vi "TriWave2ndEd_YNWang.vi"() -> ()   [LabVIEW 2014]
uses:
  <vilib>/Instr/_visa.llb/VISA Configure Serial Port (Instr).vi
panel:
  out "Measured Curr":dbl
  out "Output Volt":dbl
  out "V-I Diagram":cluster{dbl[], dbl[]}(graph)
  in  "VISA Name":refnum<visa-resource-name>
  in  "Path":path
  in  "Protect Scan":bool
  in  "Reverse?":bool
  in  "Pause":bool
  in  "stop":bool
  in  "End":dbl format="%#_13g"
  in  "Cycle":i32
  in  "milliseconds to wait":u32
  out "Output V":dbl(graph)
  in  "Init":dbl format="%#_13g"
  in  "step":dbl format="%#_13g"
  in  "Min":dbl format="%#_13g"
  in  "Max":dbl format="%#_13g"
  # "Reverse"
  # "Normal"
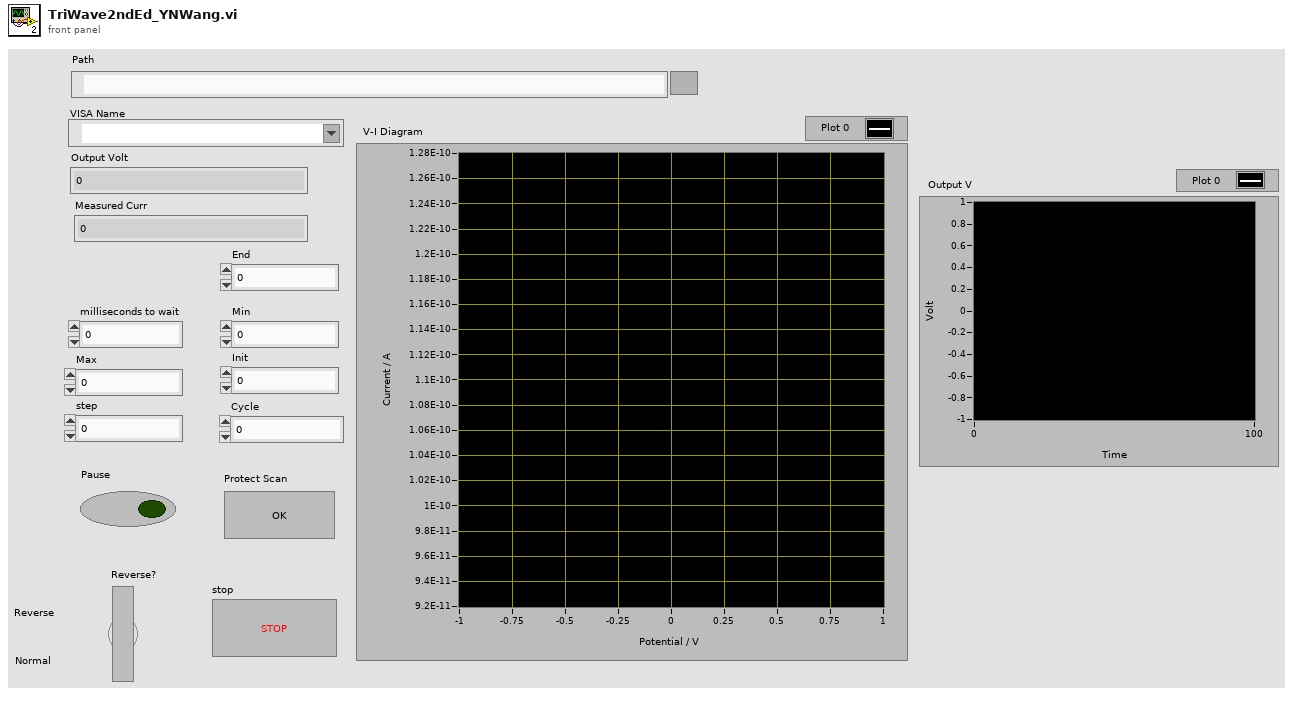
[diagram p1: front panel]
types:
  T1 = enum16{"open", "replace", "create", "open or create", "replace or create", "replace or create with confirmation"}
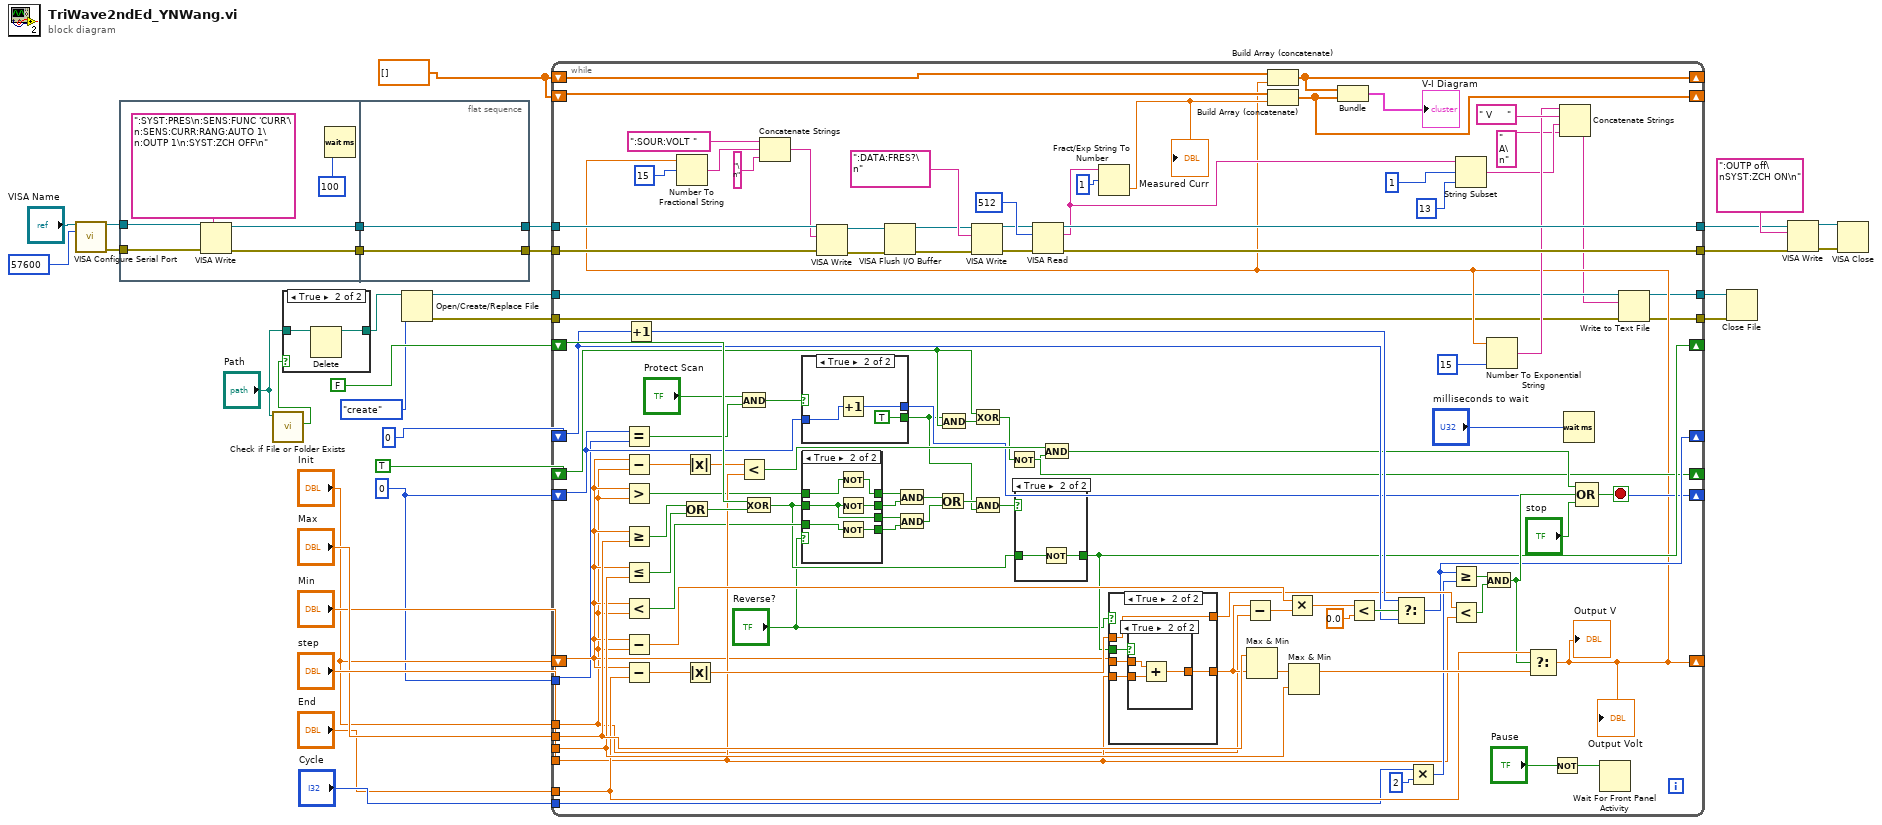
[diagram p0: block diagram]
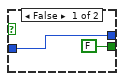
[diagram p3: hidden frame]
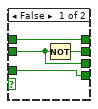
[diagram p4: hidden frame]
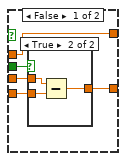
[diagram p6: hidden frame]
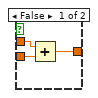
[diagram p7: hidden frame]
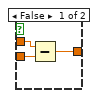
[diagram p8: hidden frame]
diagram:
  w16 = dbl[] []
  w24 = 0
  n1 = call-poly "VISA Configure Serial Port"("VISA resource name"="VISA Name", "baud rate (9600)"=57600) -> ("VISA resource name out"=w13:refnum<visa-resource-name>, "error out"=w12:errorcluster)  [unwired: 12 in]
  n2 = flat-sequence {
    tunnel: w13 -> [w38]
    tunnel: w12 -> [w37]
    tunnel: [w34] -> w4
    tunnel: [w33] -> w3
    tunnel: [w39] -> w1
    tunnel: [w40] -> w2
    tunnel: w4 -> [w40]
    tunnel: w3 -> [w39]
    frame #0 {
      n3 = VISA Write(VISA resource name=w38, write buffer=":SYST:PRES\n:SENS:FUNC 'CURR'\n:SENS:CURR:RANG:AUTO 1\n:OUTP 1\n:SYST:ZCH OFF\n", error in (no error)=w37) -> (VISA resource name out=w34:refnum<visa-resource-name>, error out=w33:errorcluster)  [unwired: 1 out]
      n4 = Wait (ms)(milliseconds to wait=u32 100) -> ()  [unwired: 1 out]
    }
    frame #1 {
    }
  }
  n5 = call <vilib>:"Check if File or Folder Exists.vi"("path"="Path") -> ("file or folder exists?"=w22:bool)  [unwired: 8 in, 2 out]
  n6 = case shown="True" w22 {
    tunnel: "Path" -> [w41 w43]
    tunnel: [w41 w42] -> w20
    frame False {
    }
    frame True {
      n7 = Delete(path (use dialog)=w43) -> (deleted path=w42:path)  [unwired: 4 in, 2 out]
    }
  }
  n8 = Open/Create/Replace File(file path (use dialog)=w20, operation (0:open)=T1."create") -> (refnum out=w18:refnum<file>, error out=w17:errorcluster)  [unwired: 4 in, 1 out]
  n9 = while {
    tunnel: "step" -> [w109]
    tunnel: "Max" -> [w139]
    tunnel: "Min" -> [w137]
    shift-right: [w112] -> _
    shift-left: FALSE -> [w142]
    shift-right: [w55] -> _
    shift-left: "Init" -> [w105]
    tunnel: "Init" -> [w104]
    shift-right: [w115] -> _
    shift-left: 0 -> [w129]
    tunnel: "Cycle" -> [w119]
    tunnel: "End" -> [w123]
    tunnel: w24 -> [w93]
    shift-right: [w95] -> _
    shift-left: w24 -> [w94]
    shift-right: [w87] -> _
    shift-left: TRUE -> [w88]
    tunnel: w18 -> [w54]
    tunnel: w17 -> [w53]
    tunnel: w2 -> [w75]
    tunnel: w1 -> [w74]
    tunnel: [w65] -> w8
    tunnel: [w64] -> w7
    tunnel: [w51] -> w6
    tunnel: [w50] -> w5
    shift-right: [w49] -> _
    shift-left: w16 -> [w81]
    shift-right: [w48] -> _
    shift-left: w16 -> [w80]
    stop <- w120 stop-if-true
    n10 = Equal?(x=w94, y=w93) -> (x = y?=w90:bool)
    n11 = Subtract(x=w105, y=w104) -> (x-y=w111:dbl)
    n12 = Greater?(x=w105, y=w104) -> (0:w100:bool)
    n13 = Greater Or Equal?(x=w105, y=w139) -> (x >= y?=w144:bool)
    n14 = Less Or Equal?(x=w105, y=w137) -> (x <= y?=w143:bool)
    n15 = Less?(x=w105, y=w104) -> (x < y?=w101:bool)
    n16 = Subtract(x=w105, y=w104) -> (x-y=w134:dbl)
    n17 = Subtract(x=w105, y=w123) -> (x-y=w128:dbl)
    n18 = Increment(x=w129) -> (x+1=w130:i32)
    n19 = Or(x=w144, y=w143) -> (x .or. y?=w141:bool)
    n20 = Absolute Value(x=w111) -> (abs(x)=w110:dbl)
    n21 = Absolute Value(x=w128) -> (abs(x)=w127:dbl)
    n22 = And(x="Protect Scan", y=w90) -> (x .and. y?=w92:bool)
    n23 = Less?(x=w110, y=w109) -> (x < y?=w108:bool)
    n24 = Exclusive Or(1:w141, 2:w142) -> (0:w98:bool)
    n25 = case shown="True" w92 {
      tunnel: [FALSE TRUE] -> w85
      tunnel: w94 -> [w145 w148]
      tunnel: [w145 w147] -> w95
      frame False {
      }
      frame True {
        n26 = Increment(x=w148) -> (x+1=w147:i32)
      }
    }
    n27 = case shown="True" "Reverse?" {
      tunnel: w101 -> [w152 w157]
      tunnel: w98 -> [w150 w154]
      tunnel: w100 -> [w153 w159]
      tunnel: [w153 w158] -> w99
      tunnel: [w152 w156] -> w83
      tunnel: [w150 w154] -> w84
      tunnel: [w151 w155] -> w82
      frame False {
        n28 = Not(x=w150) -> (.not. x?=w151:bool)
      }
      frame True {
        n29 = Not(x=w159) -> (.not. x?=w158:bool)
        n30 = Not(x=w154) -> (.not. x?=w155:bool)
        n31 = Not(x=w157) -> (.not. x?=w156:bool)
      }
    }
    n32 = And(x=w99, y=w82) -> (x .and. y?=w106:bool)
    n33 = And(x=w84, y=w83) -> (x .and. y?=w103:bool)
    n34 = Or(x=w106, y=w103) -> (x .or. y?=w97:bool)
    n35 = And(x=w85, y=w88) -> (x .and. y?=w89:bool)
    n36 = Exclusive Or(1:w89, 2:w88) -> (0:w87:bool)
    n37 = And(x=w97, y=w85) -> (x .and. y?=w102:bool)
    n38 = Not(x=w87) -> (.not. x?=w86:bool)
    n39 = case shown="True" w102 {
      tunnel: w98 -> [w160 w161]
      tunnel: [w160 w162] -> w112
      frame False {
      }
      frame True {
        n40 = Not(x=w161) -> (.not. x?=w162:bool)
      }
    }
    n41 = And(x=w108, y=w86) -> (x .and. y?=w107:bool)
    n42 = case shown="True" "Reverse?" {
      tunnel: w109 -> [w165 w176]
      tunnel: w105 -> [w166 w177]
      tunnel: [w164 w175] -> w136
      tunnel: w127 -> [w163 w174]
      tunnel: [w163 w174] -> w126
      tunnel: w112 -> [w167 w178]
      frame False {
        n43 = case shown="True" w167 {
          tunnel: w166 -> [w170 w173]
          tunnel: w165 -> [w169 w172]
          tunnel: [w168 w171] -> w164
          frame False {
            n44 = Add(x=w170, y=w169) -> (x+y=w168:dbl)
          }
          frame True {
            n45 = Subtract(x=w173, y=w172) -> (x-y=w171:dbl)
          }
        }
      }
      frame True {
        n46 = case shown="True" w178 {
          tunnel: w177 -> [w181 w184]
          tunnel: w176 -> [w180 w183]
          tunnel: [w179 w182] -> w175
          frame False {
            n47 = Subtract(x=w181, y=w180) -> (x-y=w179:dbl)
          }
          frame True {
            n48 = Add(x=w184, y=w183) -> (x+y=w182:dbl)
          }
        }
      }
    }
    n49 = Subtract(x=w136, y=w104) -> (x-y=w135:dbl)
    n50 = Max & Min(x=w139, y=w136) -> (min(x,y)=w138:dbl)  [unwired: 1 out]
    n51 = Multiply(x=w134, y=w135) -> (x*y=w133:dbl)
    n52 = Max & Min(x=w138, y=w137) -> (max(x,y)=w124:dbl)  [unwired: 1 out]
    n53 = Less?(x=w133, y=0.0) -> (x < y?=w131:bool)
    n54 = Select(t=w130, s=w131, f=w129) -> (s? t:f=w115:i32)
    n55 = Multiply(x=w119, y=2) -> (x*y=w116:i32)
    n56 = Greater Or Equal?(x=w115, y=w116) -> (x >= y?=w117:bool)
    n57 = Less?(x=w126, y=w109) -> (x < y?=w125:bool)
    n58 = And(x=w117, y=w125) -> (x .and. y?=w121:bool)
    n59 = Select(t=w123, s=w121, f=w124) -> (s? t:f=w55:dbl)
    "Output V" <- w55
    "Output Volt" <- w55
    n60 = Number To Fractional String(number=w55, width (-)=15) -> (F-format string=w77:string)  [unwired: 2 in]
    n61 = Concatenate Strings(":SOUR:VOLT ", w77, "\n") -> (w73:string)
    n62 = VISA Write(VISA resource name=w75, write buffer=w73, error in (no error)=w74) -> (VISA resource name out=w47:refnum<visa-resource-name>, error out=w46:errorcluster)  [unwired: 1 out]
    n63 = VISA Flush I/O Buffer(VISA resource name=w47, error in (no error)=w46) -> (VISA resource name out=w45:refnum<visa-resource-name>, error out=w44:errorcluster)  [unwired: 1 in]
    n64 = VISA Write(VISA resource name=w45, write buffer=":DATA:FRES?\n", error in (no error)=w44) -> (VISA resource name out=w69:refnum<visa-resource-name>, error out=w68:errorcluster)  [unwired: 1 out]
    n65 = VISA Read(VISA resource name=w69, byte count=u32 512, error in (no error)=w68) -> (VISA resource name out=w65:refnum<visa-resource-name>, read buffer=w56:string, error out=w64:errorcluster)  [unwired: 1 out]
    n66 = Fract/Exp String To Number(string=w56, offset=1) -> (number=w67:dbl)  [unwired: 2 in, 1 out]
    "Measured Curr" <- w67
    n67 = Build Array (concatenate)(w81, w55) -> (w49:dbl[])
    n68 = Build Array (concatenate)(w80, w67) -> (w48:dbl[])
    n69 = Bundle(w49, w48) -> (→"V-I Diagram":cluster{dbl[], dbl[]})  [unwired: 1 in]
    n70 = String Subset(string=w56, offset (0)=1, length (rest)=13 ("length (rest)")) -> (substring=w59:string)
    n71 = Number To Exponential String(number=w55, precision (6)=15) -> (E-format string=w62:string)  [unwired: 2 in]
    n72 = Not(x="Pause") -> (.not. x?=w113:bool)
    n73 = Concatenate Strings(w62, " V     ", w59, " A\n") -> (w52:string)
    n74 = Wait (ms)(milliseconds to wait="milliseconds to wait") -> ()  [unwired: 1 out]
    n75 = Compound Arithmetic op=OR(w107, w121, "stop") -> (w120:bool)
    n76 = Wait For Front Panel Activity(3:w113) -> ()  [unwired: 2 in, 1 out]
    n77 = Write to Text File(file (use dialog)=w54, text=w52, error in=w53) -> (refnum out=w51:refnum<file>, error out=w50:errorcluster)  [unwired: 1 in, 1 out]
  }
  n78 = Close File(refnum=w6, error in=w5) -> ()  [unwired: 2 out]
  n79 = VISA Write(VISA resource name=w8, write buffer=":OUTP off\nSYST:ZCH ON\n", error in (no error)=w7) -> (VISA resource name out=w11:refnum<visa-resource-name>, error out=w10:errorcluster)  [unwired: 1 out]
  n80 = VISA Close(VISA resource name=w11, error in (no error)=w10) -> ()  [unwired: 1 out]
